vi "AssertNotEquals.vi"(5 "Expected":variant, 7 "Message (\"\")":string, 8 "error in (no error)":errorcluster, 10 "Actual":variant) -> (0 "error out":errorcluster)   [LabVIEW 2019, in "Assertion.lvlib"]
doc: "Asserts that two variables are not equal. Does nothing if an error occurred before this node runs. Returns an error if the assertion failed. Optionally adds a message to the error message if the assertion failed."
uses:
  Assertion.lvlib
  Constraint/IsEqual/IsEqual.lvclass
  Constraint/UnaryOperator/UnaryOperator.lvclass
  Constraint/LogicalNot/LogicalNot.lvclass
  C:/Users/de200256/Code/LVUnit/Constraint/Constraint/Constraint.lvclass
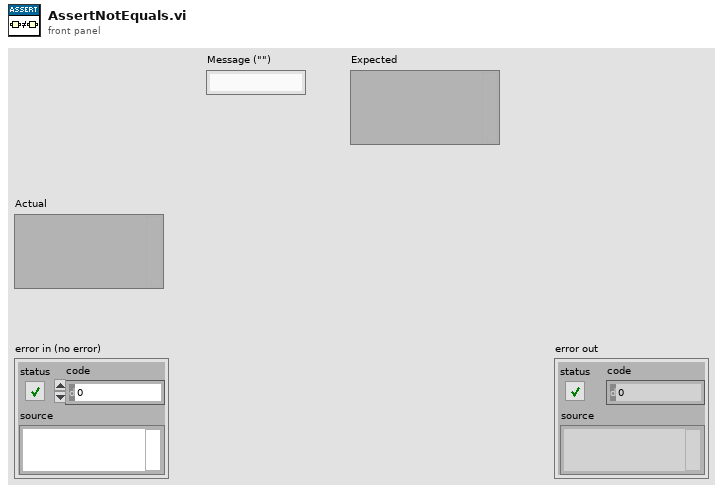
[diagram p1: front panel]
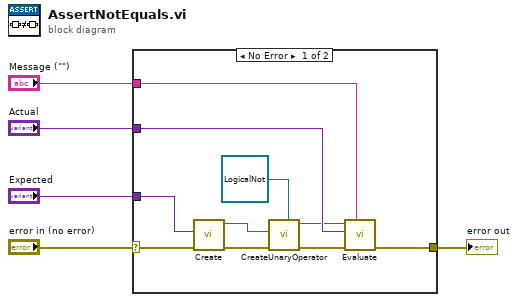
[diagram p0: block diagram]
diagram:
  n1 = case shown="No Error" "error in (no error)" {
    selector: "error in (no error)" -> [w12 w16]
    tunnel: "Actual" -> [w15 _]
    tunnel: [w14 w16] -> w4
    tunnel: "Message (\"\")" -> [w13 _]
    tunnel: "Expected" -> [w10 _]
    frame No Error {
      n2 = call "Create.vi"("error in (no error)"=w12, "Expected"=w10) -> ("error out"=w11:errorcluster, "IsEqual"=w8:refnum<class "IsEqual.lvclass">)  [unwired: 8 in]
      n3 = call-dynamic "CreateUnaryOperator.vi"("UnaryOperator In"=refnum<class "LogicalNot.lvclass"> refnum, "error in (no error)"=w11, "Constraint"=w8) -> ("error out"=w9:errorcluster, "UnaryOperator"=w7:refnum<class "UnaryOperator.lvclass">)  [unwired: 7 in]
      n4 = call-dynamic "Evaluate.vi"("Message (\"\")"=w13, "error in (no error)"=w9, "Actual"=w15, "Constraint in"=w7) -> ("error out"=w14:errorcluster)  [unwired: 6 in, 1 out]
    }
    frame Error {
    }
  }
  "error out" <- w4
